vi "CONEX-CC SubVi.vi"(0 "Connection Cluster out":T1) -> (4 "Connection Cluster out 2":T1)   [LabVIEW 2016]
doc: "CONEX - CC Virtual Front Panel:\n\nThis is a sample of an application that can be built with the LabVIEW drivers.\n\nPress HOME / ENABLE in top left of panel to put stage in Ready state for motion."
uses:
  <vilib>/Platform/TimedLoop/XDataNode/timing_clust.ctl
  <vilib>/Platform/TimedLoop/XDataNode/nitl_modes.ctl
  <vilib>/Platform/TimedLoop/XDataNode/wakeup.ctl
  <vilib>/Platform/TimedLoop/XDataNode/XDataNode.xnode
  <vilib>/Platform/TimedLoop/XDataNode/XDNodeRunTimeDep.lvlib
panel:
  out "counter":i32
  in  "Set Max":bool
  in  "Set Min":bool
  in  "Max":dbl
  in  "Min":dbl
  in  "Set velocity":bool
  out "Stop cycle":bool=TRUE
  in  "Cycle":bool
  in  "# Loops":i32=5
  in  "Go2":bool
  in  "Go1":bool
  in  "Abs. Move 2":dbl=1.0
  in  "Abs. Move 1":dbl
  in  "-":bool
  in  "+":bool
  in  "Step":dbl
  out "Position History":dbl(graph)=1.5
  in  "Action":bool
  out "Stop polling":bool=TRUE
  out "Controller state description":string="STATUS"
  out "Controller state":string="33"
  out "Positioner error":string="0000"
  in  "Velocity:":dbl
  in  "Exit":bool=TRUE
  out "Target position":dbl
  in  "Position glissière":cluster{dbl, dbl}(slide) scale=0.0..25.0
  in  "Exit":bool
  out "Current position":dbl
  # "unit/s"
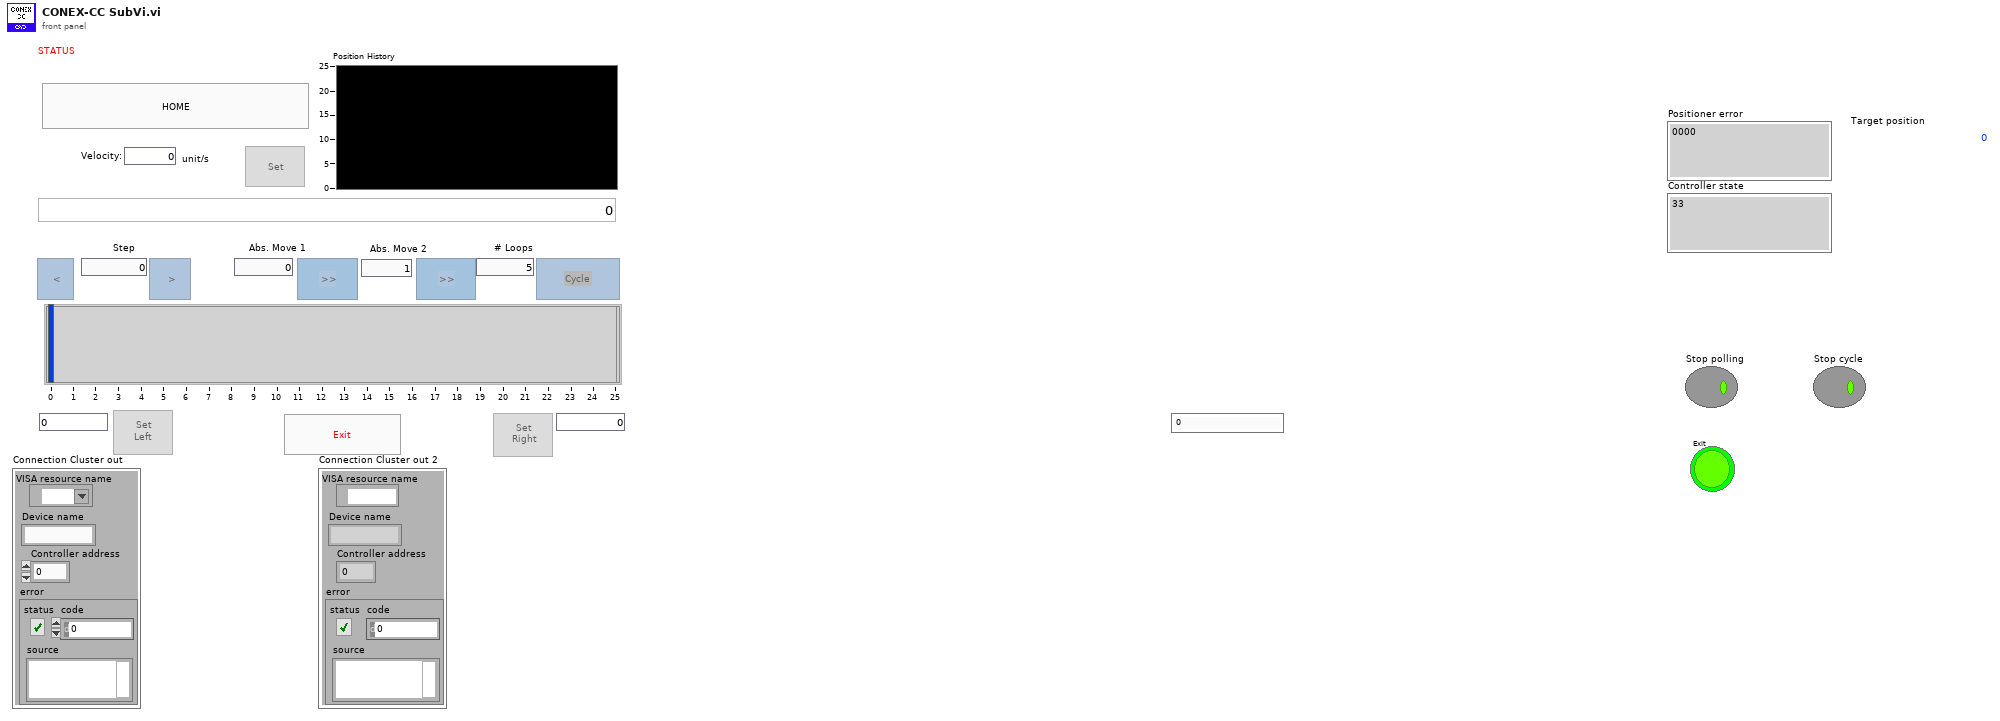
[diagram p1: front panel]
types:
  T1 = cluster{"VISA resource name":refnum<visa-resource-name>, "Device name":string, "Controller address":i32, "error":errorcluster}
  T2 = typedef "XDNodeRunTimeDep.lvlib/timing_clust.ctl" = cluster{"Expected End [f-1]":u64, "Actual End [f-1]":u64, "Finished Late? [f-1]":bool, "Expected End [i-1]":u64, "Actual End [i-1]":u64, "Finished Late? [i-1]":bool, "Expected Start [i]":u64, "Actual Start [i]":u64, "Expected Start [f]":u64, "Actual Start [f]":u64, "Source Name":string, "Structure Name":string, "Period":i64, "Deadline":i64, "Offset":i64, "Start":i64, "Priority":i32, "Timeout":i32, "Mode":T3, "Wakeup Reason":T4, "Error":errorcluster, "Source Type":string, "Secondary Source Type":string, "Global End Time":u64, "Global Start Time":u64, "Frame Duration":u64, "Iteration Duration":u64, "Assigned CPU":i32, "I/O Scan Engine Mode":u32}
  T3 = typedef "XDNodeRunTimeDep.lvlib/nitl_modes.ctl" = enum32{"No Change", "Process missed periods, maintain original phase", "Discard missed periods, maintain original phase", "Process missed periods, ignore original phase", "Discard missed periods, ignore original phase"}
  T4 = typedef "XDNodeRunTimeDep.lvlib/wakeup.ctl" = enum32{"Normal", "Aborted", "Asynchronous wakeup", "Timing source error", "Timed loop error", "Timeout"}
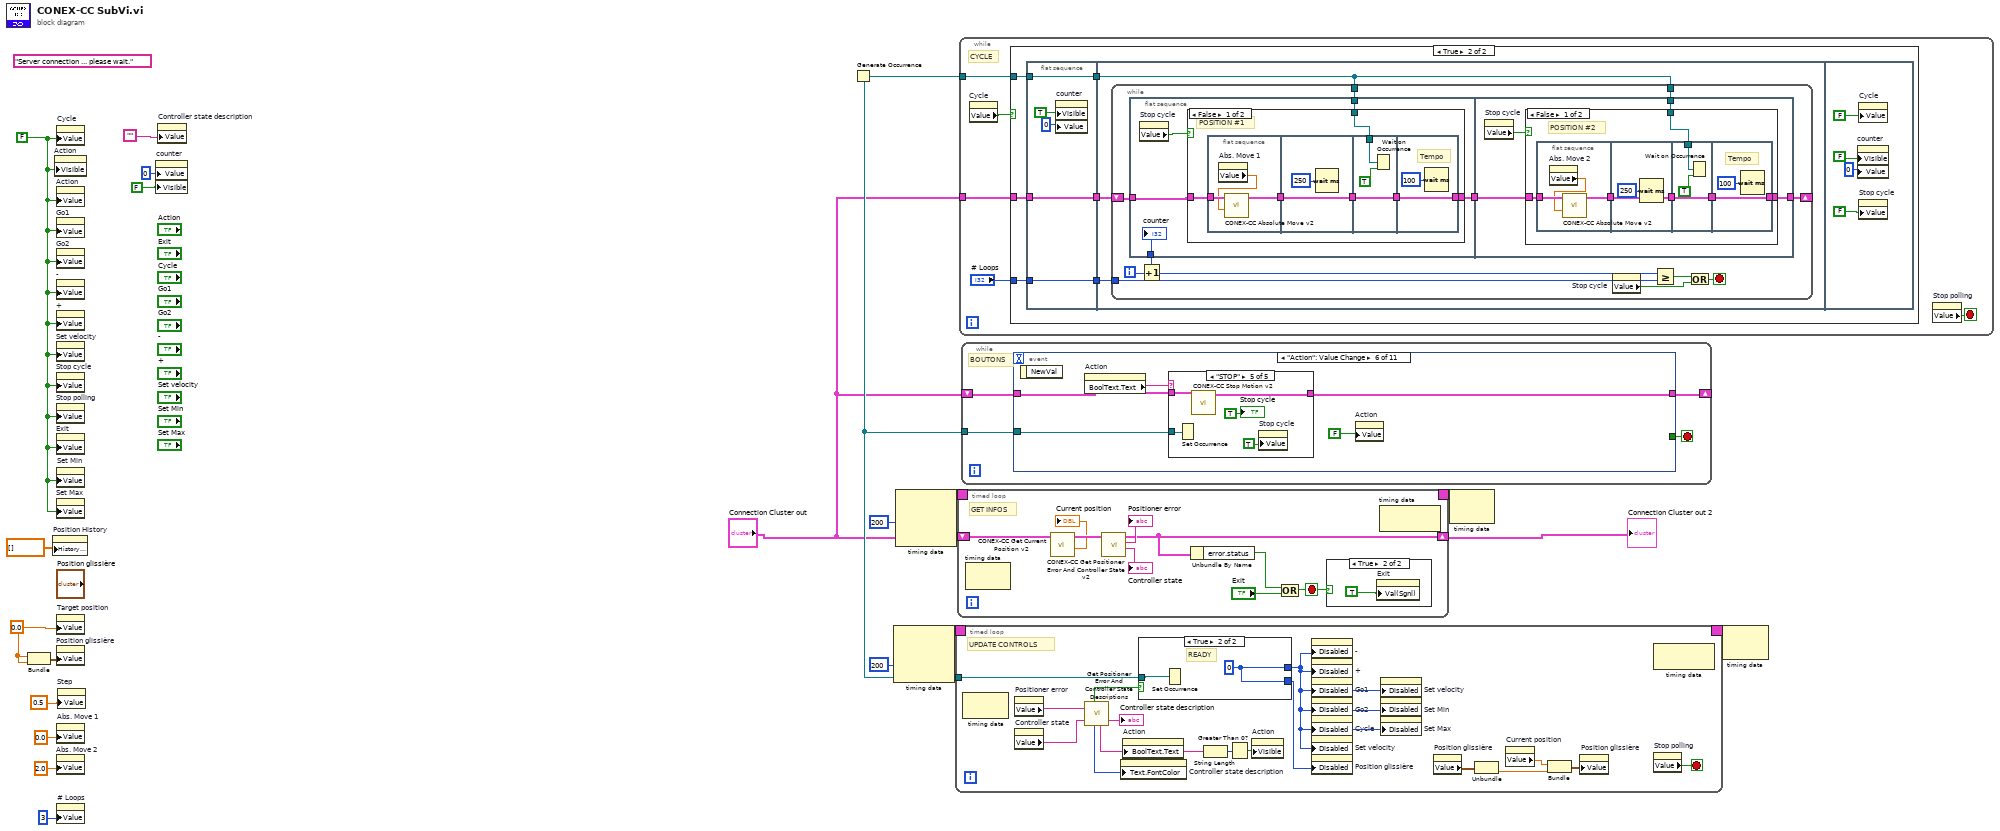
[diagram p0: block diagram]
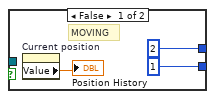
[diagram p5: hidden frame]
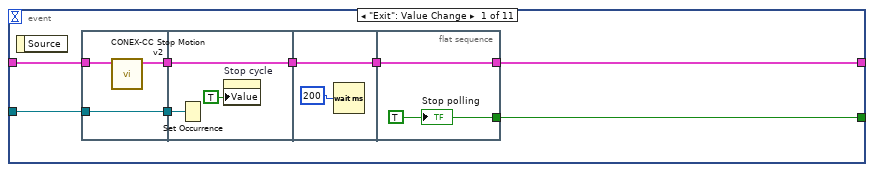
[diagram p6: hidden frame]
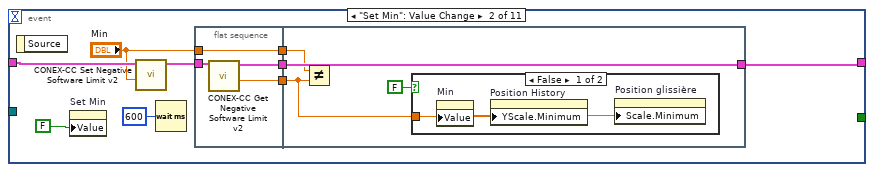
[diagram p7: hidden frame]
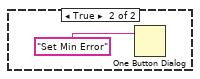
[diagram p8: hidden frame]
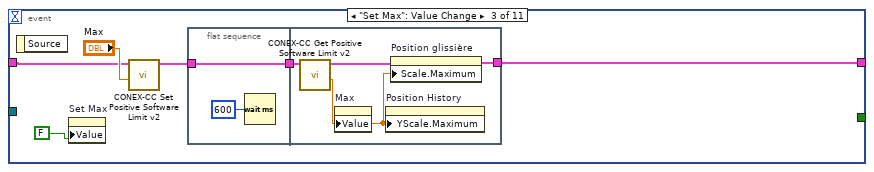
[diagram p9: hidden frame]
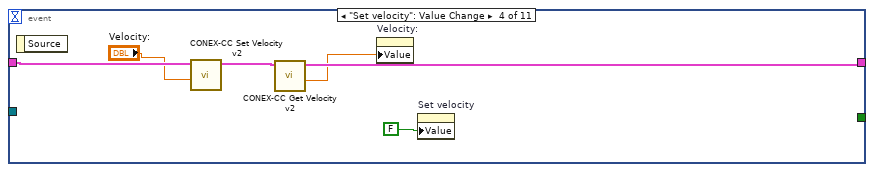
[diagram p10: hidden frame]
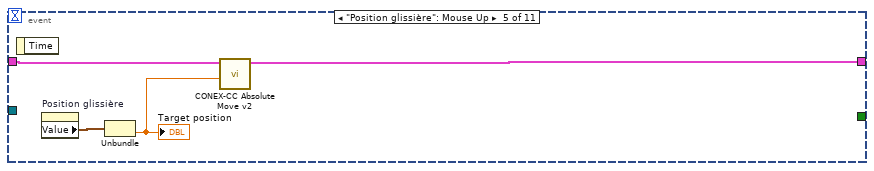
[diagram p11: hidden frame]
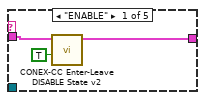
[diagram p12: hidden frame]
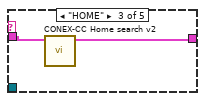
[diagram p14: hidden frame]
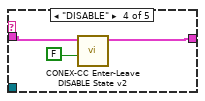
[diagram p15: hidden frame]
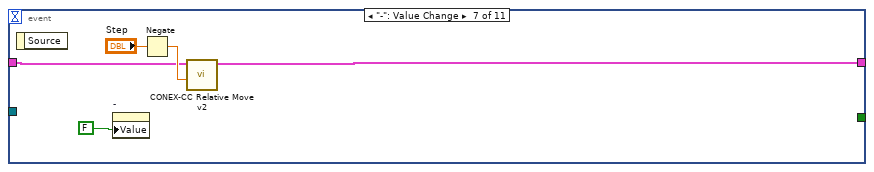
[diagram p16: hidden frame]
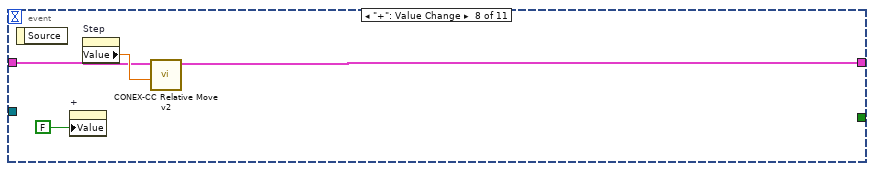
[diagram p17: hidden frame]
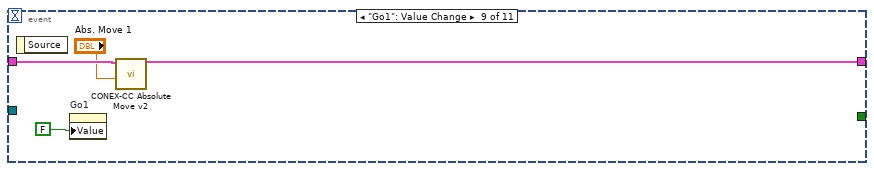
[diagram p18: hidden frame]
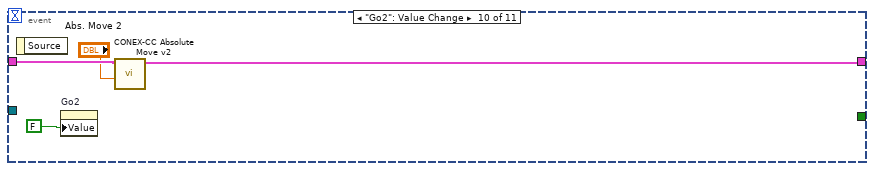
[diagram p19: hidden frame]
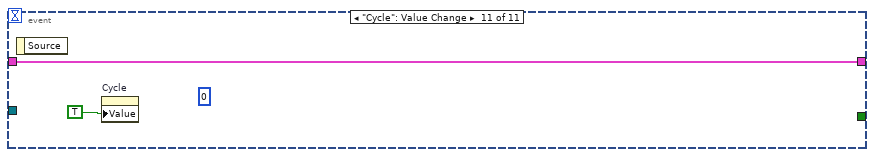
[diagram p20: hidden frame]
diagram:
  (unwired) "Server connection ... please wait." ("Title")
  w16 = FALSE
  w19 = 0.0
  n1 = Bundle(w19, w19) -> (w20:cluster{dbl, dbl})  [unwired: 1 out]
  n2 = property on="Position History" class="WFChart (strict)"("History Data"=dbl[] [] ("Données d'historique")) -> ()  [unwired: 2 in, 2 out]
  n3 = property on="Action" class="Bool (strict)"("Visible"=w16) -> ()  [unwired: 2 in, 2 out]
  n4 = property on="Cycle" class="Bool (strict)"("Value"=w16) -> ()  [unwired: 2 in, 2 out]
  n5 = property on="Action" class="Bool (strict)"("Value"=w16) -> ()  [unwired: 2 in, 2 out]
  n6 = property on="Go1" class="Bool (strict)"("Value"=w16) -> ()  [unwired: 2 in, 2 out]
  n7 = property on="Go2" class="Bool (strict)"("Value"=w16) -> ()  [unwired: 2 in, 2 out]
  n8 = property on="-" class="Bool (strict)"("Value"=w16) -> ()  [unwired: 2 in, 2 out]
  n9 = property on="+" class="Bool (strict)"("Value"=w16) -> ()  [unwired: 2 in, 2 out]
  n10 = property on="Set velocity" class="Bool (strict)"("Value"=w16) -> ()  [unwired: 2 in, 2 out]
  n11 = property on="Stop cycle" class="Bool (strict)"("Value"=w16) -> ()  [unwired: 2 in, 2 out]
  n12 = property on="Stop polling" class="Bool (strict)"("Value"=w16) -> ()  [unwired: 2 in, 2 out]
  n13 = property on="Exit" class="Bool (strict)"("Value"=w16) -> ()  [unwired: 2 in, 2 out]
  n14 = property on="Set Min" class="Bool (strict)"("Value"=w16) -> ()  [unwired: 2 in, 2 out]
  n15 = property on="Set Max" class="Bool (strict)"("Value"=w16) -> ()  [unwired: 2 in, 2 out]
  n16 = property on="Target position" class="DigNum (strict)"("Value"=w19) -> ()  [unwired: 2 in, 2 out]
  n17 = property on="Position glissière" class="Slide (strict)"("Value"=w20) -> ()  [unwired: 2 in, 2 out]
  n18 = property on="Abs. Move 1" class="DigNum (strict)"("Value"=0.0 ("Abs. Move 1")) -> ()  [unwired: 2 in, 2 out]
  n19 = property on="Abs. Move 2" class="DigNum (strict)"("Value"=2.0 ("Abs. Move 2")) -> ()  [unwired: 2 in, 2 out]
  n20 = property on="# Loops" class="DigNum (strict)"("Value"=3 ("# Loops")) -> ()  [unwired: 2 in, 2 out]
  n21 = property on="Step" class="DigNum (strict)"("Value"=0.5 ("Step")) -> ()  [unwired: 2 in, 2 out]
  n22 = property on="counter" class="DigNum (strict)"("Value"=0 ("counter"), "Visible"=FALSE) -> ()  [unwired: 2 in, 2 out]
  n23 = property on="Controller state description" class="Str"("Value"="") -> ()  [unwired: 2 in, 2 out]
  n24 = Generate Occurrence() -> (w3:refnum<k4>)
  n25 = node-c288(i64 200 ("Période")) -> (w7:T2)  [unwired: 1 in, 1 out]
  n26 = node-c288(i64 200 ("Période")) -> (w9:T2)  [unwired: 1 in, 1 out]
  n27 = timed-loop {
    timing: w7 -> [_]
    timing-out: [_] -> w6
    tunnel: w3 -> [w25]
    stop <- w27 stop-if-true
    # "UPDATE CONTROLS"
    n28 = node-c288() -> ()  [unwired: 2 out]
    n29 = property on="Positioner error" class="Str"() -> ("Value"=w36:string)  [unwired: 2 in, 2 out]
    n30 = property on="Controller state" class="Str"() -> ("Value"=w35:string)  [unwired: 2 in, 2 out]
    n31 = call <userlib>:"Get Positioner Error And Controller State Descriptions.vi"("Controller state"=w35, "Positioner error"=w36) -> ("Color"=w33:u32, "Action name"=w32:string, "Controller state description"=→"Controller state description":string, "IsReady?"=w29:bool)  [unwired: 2 out]
    n32 = property on="Controller state description" class="Str"("Text.FontColor"=w33) -> ()  [unwired: 2 in, 2 out]
    n33 = property on="Action" class="Bool (strict)"("BoolText.Text"=w32) -> ()  [unwired: 2 in, 2 out]
    n34 = case shown="True" w29 {
      tunnel: [u8 2 w41] -> w26
      tunnel: [u8 1 w41] -> w28
      tunnel: w25 -> [_ w40]
      frame False {
        # "MOVING"
        n35 = property on="Current position" class="DigNum (strict)"() -> ("Value"=→"Position History":dbl)  [unwired: 2 in, 2 out]
      }
      frame True {
        w41 = u8 0
        # "READY"
        n36 = Set Occurrence(w40) -> ()
      }
    }
    n37 = String Length(string=w32) -> (length=w31:i32)
    n38 = Greater Than 0?(x=w31) -> (x > 0?=w30:bool)
    n39 = property on="Action" class="Bool (strict)"("Visible"=w30) -> ()  [unwired: 2 in, 2 out]
    n40 = property on="-" class="Bool (strict)"("Disabled"=w26) -> ()  [unwired: 2 in, 2 out]
    n41 = property on="+" class="Bool (strict)"("Disabled"=w26) -> ()  [unwired: 2 in, 2 out]
    n42 = property on="Go1" class="Bool (strict)"("Disabled"=w26) -> ()  [unwired: 2 in, 2 out]
    n43 = property on="Go2" class="Bool (strict)"("Disabled"=w26) -> ()  [unwired: 2 in, 2 out]
    n44 = property on="Cycle" class="Bool (strict)"("Disabled"=w26) -> ()  [unwired: 2 in, 2 out]
    n45 = property on="Set velocity" class="Bool (strict)"("Disabled"=w26) -> ()  [unwired: 2 in, 2 out]
    n46 = property on="Position glissière" class="Slide (strict)"("Disabled"=w28) -> ()  [unwired: 2 in, 2 out]
    n47 = property on="Set velocity" class="Bool (strict)"("Disabled"=w26) -> ()  [unwired: 2 in, 2 out]
    n48 = property on="Set Min" class="Bool (strict)"("Disabled"=w26) -> ()  [unwired: 2 in, 2 out]
    n49 = property on="Set Max" class="Bool (strict)"("Disabled"=w26) -> ()  [unwired: 2 in, 2 out]
    n50 = property on="Position glissière" class="Slide (strict)"() -> ("Value"=w22:cluster{dbl, dbl})  [unwired: 2 in, 2 out]
    n51 = Unbundle(w22) -> (w21:dbl)  [unwired: 1 out]
    n52 = property on="Current position" class="DigNum (strict)"() -> ("Value"=w23:dbl)  [unwired: 2 in, 2 out]
    n53 = Bundle("Value"=w23, w21) -> (w24:cluster{"Value":dbl, dbl})  [unwired: 1 out]
    n54 = property on="Position glissière" class="Slide (strict)"("Value"=w24) -> ()  [unwired: 2 in, 2 out]
    n55 = node-c288() -> ()  [unwired: 2 out]
    n56 = property on="Stop polling" class="Bool (strict)"() -> ("Value"=w27:bool)  [unwired: 2 in, 2 out]
  }
  n57 = timed-loop {
    timing: w9 -> [_]
    timing-out: [_] -> w8
    shift-right: [w46] -> w1
    shift-left: "Connection Cluster out" -> [w48]
    stop <- w50 stop-if-true
    # "GET INFOS"
    n58 = node-c288() -> ()  [unwired: 2 out]
    n59 = call <userlib>:"CONEX-CC Get Current Position v2.vi"("Connection Cluster in"=w48) -> ("Current position"=→"Current position":dbl, "Connection Cluster out"=w47:T1)  [unwired: 8 in, 1 out]
    n60 = call <userlib>:"CONEX-CC Get Positioner Error And Controller State v2.vi"("Connection Cluster in"=w47) -> ("Controller state"=→"Controller state":string, "Positioner error"=→"Positioner error":string, "Connection Cluster out"=w46:T1)  [unwired: 8 in]
    n61 = Unbundle By Name(w46) -> ("error.status"=w45:bool)
    n62 = Or(x=w45, y="Exit") -> (x .or. y?=w50:bool)
    n63 = case shown="True" w50 {
      frame False {
      }
      frame True {
        n64 = property on="Exit" class="Bool (strict)"("Val(Sgnl)"=TRUE) -> ()  [unwired: 2 in, 2 out]
      }
    }
    n65 = node-c288() -> ()  [unwired: 2 out]
  }
  "Connection Cluster out 2" <- w1
  n66 = while {
    tunnel: "Connection Cluster out" -> [w60]
    tunnel: w3 -> [w56]
    stop <- w59 stop-if-true
    # "CYCLE"
    n67 = property on="Cycle" class="Bool (strict)"() -> ("Value"=w58:bool)  [unwired: 2 in, 2 out]
    n68 = case shown="True" w58 {
      tunnel: w60 -> [_ w66]
      tunnel: "# Loops" -> [_ w65]
      tunnel: w56 -> [_ w62]
      frame False {
      }
      frame True {
        n69 = flat-sequence {
          tunnel: w65 -> [w70]
          tunnel: w66 -> [w71]
          tunnel: [w71] -> w64
          tunnel: [w70] -> w63
          tunnel: w62 -> [w67]
          tunnel: [w67] -> w61
          tunnel: w64 -> [w72]
          tunnel: w63 -> [w74]
          tunnel: w61 -> [w73]
          frame #0 {
            n70 = property on="counter" class="DigNum (strict)"("Visible"=TRUE, "Value"=0 ("counter")) -> ()  [unwired: 2 in, 2 out]
          }
          frame #1 {
            n71 = while {
              tunnel: w74 -> [w85]
              shift-right: [w75] -> _
              shift-left: w72 -> [w76]
              tunnel: w73 -> [w81]
              tunnel: w73 -> [w80]
              i -> [w79]
              stop <- w84 stop-if-true
              n72 = flat-sequence {
                tunnel: [w90] -> w77
                tunnel: w81 -> [w88]
                tunnel: w78 -> [w87]
                tunnel: w76 -> [w86]
                tunnel: w77 -> [w111]
                tunnel: w80 -> [w109]
                tunnel: [w108] -> w75
                frame #0 {
                  n73 = property on="Stop cycle" class="Bool (strict)"() -> ("Value"=w89:bool)  [unwired: 2 in, 2 out]
                  n74 = case shown="False" w89 {
                    tunnel: w86 -> [w96 w107]
                    tunnel: [w95 w107] -> w90
                    tunnel: w88 -> [w94 _]
                    frame False {
                      # "POSITION #1"
                      n75 = flat-sequence {
                        tunnel: w96 -> [w98]
                        tunnel: [w99] -> w93
                        tunnel: w93 -> [w101]
                        tunnel: [w101] -> w92
                        tunnel: w92 -> [w104]
                        tunnel: w94 -> [w102]
                        tunnel: [w104] -> w91
                        tunnel: [w106] -> w95
                        tunnel: w91 -> [w106]
                        frame #0 {
                          n76 = property on="Abs. Move 1" class="DigNum (strict)"() -> ("Value"=w97:dbl)  [unwired: 2 in, 2 out]
                          n77 = call <userlib>:"CONEX-CC Absolute Move v2.vi"("Target position"=w97, "Connection Cluster in"=w98) -> ("Connection Cluster out"=w99:T1)  [unwired: 5 in, 2 out]
                        }
                        frame #1 {
                          n78 = Wait (ms)(milliseconds to wait=u32 250 ("attente (ms)")) -> ()  [unwired: 1 out]
                        }
                        frame #2 {
                          n79 = Wait on Occurrence(1:TRUE ("ignorer les précédents (V)"), 2:w102) -> ()  [unwired: 1 in, 1 out]
                        }
                        frame #3 {
                          # "Tempo"
                          n80 = Wait (ms)(milliseconds to wait=u32 100 ("attente (ms)")) -> ()  [unwired: 1 out]
                        }
                      }
                    }
                    frame True {
                    }
                  }
                  "counter" <- w87
                }
                frame #1 {
                  n81 = property on="Stop cycle" class="Bool (strict)"() -> ("Value"=w110:bool)  [unwired: 2 in, 2 out]
                  n82 = case shown="False" w110 {
                    tunnel: w111 -> [w117 w128]
                    tunnel: w109 -> [w116 _]
                    tunnel: [w115 w128] -> w108
                    frame False {
                      # "POSITION #2"
                      n83 = flat-sequence {
                        tunnel: w117 -> [w120]
                        tunnel: [w119] -> w112
                        tunnel: [w121] -> w113
                        tunnel: w112 -> [w121]
                        tunnel: w116 -> [w125]
                        tunnel: [w123] -> w114
                        tunnel: w113 -> [w123]
                        tunnel: [w126] -> w115
                        tunnel: w114 -> [w126]
                        frame #0 {
                          n84 = property on="Abs. Move 2" class="DigNum (strict)"() -> ("Value"=w118:dbl)  [unwired: 2 in, 2 out]
                          n85 = call <userlib>:"CONEX-CC Absolute Move v2.vi"("Target position"=w118, "Connection Cluster in"=w120) -> ("Connection Cluster out"=w119:T1)  [unwired: 5 in, 2 out]
                        }
                        frame #1 {
                          n86 = Wait (ms)(milliseconds to wait=u32 250 ("attente (ms)")) -> ()  [unwired: 1 out]
                        }
                        frame #2 {
                          n87 = Wait on Occurrence(1:TRUE ("ignorer les précédents (V)"), 2:w125) -> ()  [unwired: 1 in, 1 out]
                        }
                        frame #3 {
                          # "Tempo"
                          n88 = Wait (ms)(milliseconds to wait=u32 100 ("attente (ms)")) -> ()  [unwired: 1 out]
                        }
                      }
                    }
                    frame True {
                    }
                  }
                }
              }
              n89 = Increment(x=w79) -> (x+1=w78:i32)
              n90 = property on="Stop cycle" class="Bool (strict)"() -> ("Value"=w82:bool)  [unwired: 2 in, 2 out]
              n91 = Greater Or Equal?(x=w78, y=w85) -> (x >= y?=w83:bool)
              n92 = Or(x=w83, y=w82) -> (x .or. y?=w84:bool)
            }
          }
          frame #2 {
            n93 = property on="counter" class="DigNum (strict)"("Visible"=FALSE, "Value"=0 ("counter")) -> ()  [unwired: 2 in, 2 out]
            n94 = property on="Cycle" class="Bool (strict)"("Value"=FALSE ("Cycle")) -> ()  [unwired: 2 in, 2 out]
            n95 = property on="Stop cycle" class="Bool (strict)"("Value"=FALSE ("Cycle")) -> ()  [unwired: 2 in, 2 out]
          }
        }
      }
    }
    n96 = property on="Stop polling" class="Bool (strict)"() -> ("Value"=w59:bool)  [unwired: 2 in, 2 out]
  }
  n97 = while {
    shift-right: [w136] -> _
    shift-left: "Connection Cluster out" -> [w135]
    tunnel: w3 -> [w133]
    stop <- w134 stop-if-true
    # "BOUTONS"
    n98 = event shown="[5] \"Action\": Value Change" {
      selector: _ -> [_ _ _ _ _ _ _ _ _ _ _]
      dyn-events: _ -> [_ _ _ _ _ _ _ _ _ _ _]
      timeout: _ -> [_ _ _ _ _ _ _ _ _ _ _]
      tunnel: [w142 _ _ _ _ _ _ _ _ _ _] -> w134
      tunnel: w135 -> [w137 w161 w175 w187 w193 w198 w214 w220 w225 w229 w231]
      tunnel: [w144 w160 w174 w190 w192 w197 w218 w219 w223 w228 w231] -> w136
      tunnel: w133 -> [w139 _ _ _ _ w195 _ _ _ _ _]
      event "Exit": Value Change {
        n99 = event-data() -> ()  [unwired: 2 out]
        n100 = flat-sequence {
          tunnel: [w147] -> w143
          tunnel: w139 -> [w146]
          tunnel: [w146] -> w138
          tunnel: w137 -> [w145]
          tunnel: w143 -> [w150]
          tunnel: [w150] -> w141
          tunnel: w138 -> [w148]
          tunnel: w141 -> [w152]
          tunnel: [w152] -> w140
          tunnel: [w154] -> w144
          tunnel: w140 -> [w154]
          tunnel: [w153] -> w142
          frame #0 {
            n101 = call <userlib>:"CONEX-CC Stop Motion v2.vi"("Connection Cluster in"=w145) -> ("Connection Cluster out"=w147:T1)  [unwired: 10 in]
          }
          frame #1 {
            n102 = Set Occurrence(w148) -> ()
            n103 = property on="Stop cycle" class="Bool (strict)"("Value"=TRUE) -> ()  [unwired: 2 in, 2 out]
          }
          frame #2 {
            n104 = Wait (ms)(milliseconds to wait=u32 200 ("attente (ms)")) -> ()  [unwired: 1 out]
          }
          frame #3 {
            w153 = TRUE
            "Stop polling" <- w153
          }
        }
      }
      event "Set Min": Value Change {
        n105 = event-data() -> ()  [unwired: 2 out]
        n106 = property on="Set Min" class="Bool (strict)"("Value"=FALSE ("Set Min")) -> ()  [unwired: 2 in, 2 out]
        n107 = call <userlib>:"CONEX-CC Set Negative Software Limit v2.vi"("Negative limit (left)"="Min", "Connection Cluster in"=w161) -> ("Connection Cluster out"=w163:T1)  [unwired: 9 in]
        n108 = Wait (ms)(milliseconds to wait=u32 600 ("attente (ms)")) -> ()  [unwired: 1 out]
        n109 = flat-sequence {
          tunnel: w163 -> [w167]
          tunnel: [w166] -> w158
          tunnel: [w165] -> w157
          tunnel: "Min" -> [w165]
          tunnel: [w164] -> w155
          tunnel: [w171] -> w160
          tunnel: w158 -> [w171]
          tunnel: w157 -> [w170]
          tunnel: w155 -> [w168]
          frame #0 {
            n110 = call <userlib>:"CONEX-CC Get Negative Software Limit v2.vi"("Connection Cluster in"=w167) -> ("Left limit"=w164:dbl, "Connection Cluster out"=w166:T1)  [unwired: 9 in]
          }
          frame #1 {
            n111 = Not Equal?(x=w170, y=w168) -> ()  [unwired: 1 out]
            n112 = case shown="False" FALSE {
              tunnel: w168 -> [w172 _]
              frame False {
                n113 = property on="Min" class="DigNum (strict)"("Value"=w172) -> ()  [unwired: 2 in, 2 out]
                n114 = property on="Position History" class="WFChart (strict)"("YScale.Minimum"=w172) -> ()  [unwired: 2 in, 2 out]
                n115 = property on="Position glissière" class="Slide (strict)"("Scale.Minimum"=w172) -> ()  [unwired: 2 in, 2 out]
              }
              frame True {
                n116 = One Button Dialog(message="Set Min Error") -> ()  [unwired: 1 in, 1 out]
              }
            }
          }
        }
      }
      event "Set Max": Value Change {
        n117 = event-data() -> ()  [unwired: 2 out]
        n118 = property on="Set Max" class="Bool (strict)"("Value"=FALSE ("Set Max")) -> ()  [unwired: 2 in, 2 out]
        n119 = call <userlib>:"CONEX-CC Set Positive Software Limit v2.vi"("Positive limit (right)"="Max", "Connection Cluster in"=w175) -> ("Connection Cluster out"=w179:T1)  [unwired: 9 in]
        n120 = flat-sequence {
          tunnel: w179 -> [w181]
          tunnel: [w181] -> w176
          tunnel: [w184] -> w174
          tunnel: w176 -> [w182]
          frame #0 {
            n121 = Wait (ms)(milliseconds to wait=u32 600 ("attente (ms)")) -> ()  [unwired: 1 out]
          }
          frame #1 {
            n122 = call <userlib>:"CONEX-CC Get Positive Software Limit v2.vi"("Connection Cluster in"=w182) -> ("Right limit"=w183:dbl, "Connection Cluster out"=w184:T1)  [unwired: 9 in]
            n123 = property on="Max" class="DigNum (strict)"("Value"=w183) -> ()  [unwired: 2 in, 2 out]
            n124 = property on="Position History" class="WFChart (strict)"("YScale.Maximum"=w183) -> ()  [unwired: 2 in, 2 out]
            n125 = property on="Position glissière" class="Slide (strict)"("Scale.Maximum"=w183) -> ()  [unwired: 2 in, 2 out]
          }
        }
      }
      event "Set velocity": Value Change {
        n126 = event-data() -> ()  [unwired: 2 out]
        n127 = call <userlib>:"CONEX-CC Set Velocity v2.vi"("Velocity"="Velocity:", "Connection Cluster in"=w187) -> ("Connection Cluster out"=w186:T1)  [unwired: 9 in]
        n128 = call <userlib>:"CONEX-CC Get Velocity v2.vi"("Connection Cluster in"=w186) -> ("Velocity"=w189:dbl, "Connection Cluster out"=w190:T1)  [unwired: 8 in, 1 out]
        n129 = property on="Velocity:" class="DigNum (strict)"("Value"=w189) -> ()  [unwired: 2 in, 2 out]
        n130 = property on="Set velocity" class="Bool (strict)"("Value"=FALSE ("Set velocity")) -> ()  [unwired: 2 in, 2 out]
      }
      event "Position glissière": Mouse Up {
        n131 = event-data() -> ()  [unwired: 2 out]
        n132 = property on="Position glissière" class="Slide (strict)"() -> ("Value"=w194:cluster{dbl, dbl})  [unwired: 2 in, 2 out]
        n133 = Unbundle(w194) -> (w191:dbl)  [unwired: 1 out]
        "Target position" <- w191
        n134 = call <userlib>:"CONEX-CC Absolute Move v2.vi"("Target position"=w191, "Connection Cluster in"=w193) -> ("Connection Cluster out"=w192:T1)  [unwired: 5 in, 2 out]
      }
      event "Action": Value Change {
        n135 = event-data() -> ()  [unwired: 2 out]
        n136 = property on="Action" class="Bool (strict)"() -> ("BoolText.Text"=w199:string)  [unwired: 2 in, 2 out]
        n137 = case shown="\"STOP\"" w199 {
          tunnel: w198 -> [w201 w203 w205 w208 w210]
          tunnel: [w200 w203 w204 w207 w213] -> w197
          tunnel: w195 -> [_ _ _ _ w211]
          frame "ENABLE" {
            n138 = call <userlib>:"CONEX-CC Enter-Leave DISABLE State v2.vi"("Ready? (false=DISABLE true=READY)"=TRUE ("Flag (false=DISABLE true=READY)"), "Connection Cluster in"=w201) -> ("Connection Cluster out"=w200:T1)  [unwired: 7 in]
          }
          frame Default {
          }
          frame "HOME" {
            n139 = call <userlib>:"CONEX-CC Home search v2.vi"("Connection Cluster in"=w205) -> ("Connection Cluster out"=w204:T1)  [unwired: 5 in, 3 out]
          }
          frame "DISABLE" {
            n140 = call <userlib>:"CONEX-CC Enter-Leave DISABLE State v2.vi"("Ready? (false=DISABLE true=READY)"=FALSE ("Flag (false=DISABLE true=READY)"), "Connection Cluster in"=w208) -> ("Connection Cluster out"=w207:T1)  [unwired: 7 in]
          }
          frame "STOP" {
            n141 = Set Occurrence(w211) -> ()
            n142 = call <userlib>:"CONEX-CC Stop Motion v2.vi"("Connection Cluster in"=w210) -> ("Connection Cluster out"=w213:T1)  [unwired: 10 in]
            n143 = property on="Stop cycle" class="Bool (strict)"("Value"=TRUE) -> ()  [unwired: 2 in, 2 out]
            "Stop cycle" <- TRUE ("Stop cycle")
          }
        }
        n144 = property on="Action" class="Bool (strict)"("Value"=FALSE) -> ()  [unwired: 2 in, 2 out]
      }
      event "-": Value Change {
        n145 = event-data() -> ()  [unwired: 2 out]
        n146 = property on="-" class="Bool (strict)"("Value"=FALSE ("-")) -> ()  [unwired: 2 in, 2 out]
        n147 = Negate(x="Step") -> (-x=w216:dbl)
        n148 = call <userlib>:"CONEX-CC Relative Move v2.vi"("Relative displacement"=w216, "Connection Cluster in"=w214) -> ("Connection Cluster out"=w218:T1)  [unwired: 9 in]
      }
      event "+": Value Change {
        n149 = event-data() -> ()  [unwired: 2 out]
        n150 = property on="+" class="Bool (strict)"("Value"=FALSE ("+")) -> ()  [unwired: 2 in, 2 out]
        n151 = property on="Step" class="DigNum (strict)"() -> ("Value"=w222:dbl)  [unwired: 2 in, 2 out]
        n152 = call <userlib>:"CONEX-CC Relative Move v2.vi"("Relative displacement"=w222, "Connection Cluster in"=w220) -> ("Connection Cluster out"=w219:T1)  [unwired: 9 in]
      }
      event "Go1": Value Change {
        n153 = event-data() -> ()  [unwired: 2 out]
        n154 = property on="Go1" class="Bool (strict)"("Value"=FALSE ("Go1")) -> ()  [unwired: 2 in, 2 out]
        n155 = call <userlib>:"CONEX-CC Absolute Move v2.vi"("Target position"="Abs. Move 1", "Connection Cluster in"=w225) -> ("Connection Cluster out"=w223:T1)  [unwired: 5 in, 2 out]
      }
      event "Go2": Value Change {
        n156 = event-data() -> ()  [unwired: 2 out]
        n157 = property on="Go2" class="Bool (strict)"("Value"=FALSE ("Go2")) -> ()  [unwired: 2 in, 2 out]
        n158 = call <userlib>:"CONEX-CC Absolute Move v2.vi"("Target position"="Abs. Move 2", "Connection Cluster in"=w229) -> ("Connection Cluster out"=w228:T1)  [unwired: 5 in, 2 out]
      }
      event "Cycle": Value Change {
        (unwired) 0 ("Numérique")
        n159 = event-data() -> ()  [unwired: 2 out]
        n160 = property on="Cycle" class="Bool (strict)"("Value"=TRUE ("Cycle")) -> ()  [unwired: 2 in, 2 out]
      }
    }
  }
  n161 = node-c288(w8) -> ()  [unwired: 1 out]
  n162 = node-c288(w6) -> ()  [unwired: 1 out]
